vi "Get Response.vi"(8 "error in (no error)":errorcluster, 10 "Responses Config":string[][](array[string]), 11 "Request":string) -> (0 "error out":errorcluster, 3 "Response":string)   [LabVIEW 2020]
uses:
  <vilib>/regexp/Match Regular Expression.xnode
panel:
  out "element":string
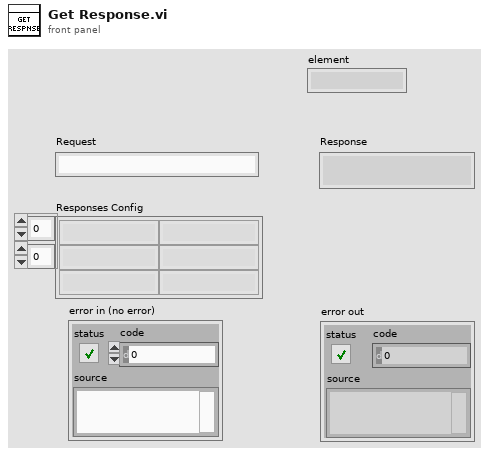
[diagram p1: front panel]
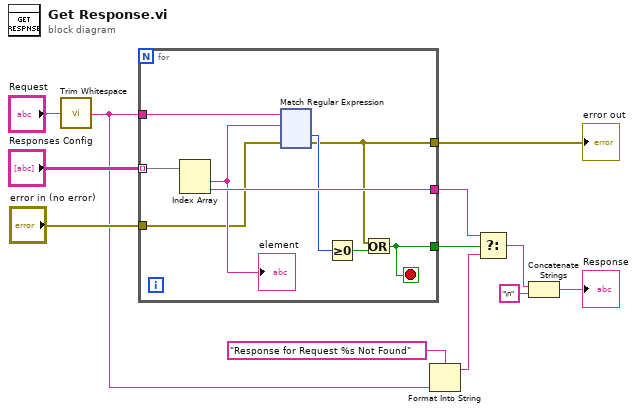
[diagram p0: block diagram]
diagram:
  n1 = call <vilib>:"Trim Whitespace.vi"("string"="Request") -> ("trimmed string"=w1:string)  [unwired: 1 in]
  n2 = for {
    tunnel: "Responses Config" -> [w21] mode=indexing
    tunnel: w1 -> [w19]
    tunnel: [w20] -> w8
    tunnel: [w15] -> w11
    tunnel: "error in (no error)" -> [w14]
    tunnel: [w13] -> w9
    stop <- w13 stop-if-true
    n3 = Index Array(array=w21) -> (element #1=w18:string, element #2=w20:string)  [unwired: 2 in]
    "element" <- w18
    n4 = xnode "Match Regular Expression"("input string"=w19, "regular expression"=w18, "error in"=w14) -> ("offset past match"=w16:i32, "error out"=w15:errorcluster)  [unwired: 3 in, 3 out]
    n5 = Greater Or Equal To 0?(x=w16) -> (x >= 0?=w17:bool)
    n6 = Or(x=w15, y=w17) -> (x .or. y?=w13:bool)
  }
  "error out" <- w11
  n7 = Format Into String(format string="Response for Request %s Not Found" ("f"), w1) -> (resulting string=w3:string)  [unwired: 2 in, 1 out]
  n8 = Select(t=w8, s=w9, f=w3) -> (s? t:f=w7:string)
  n9 = Concatenate Strings(w7, "\n" ("string")) -> (→"Response":string)
